vi "Create Dense Cell.vi"() -> ()   [LabVIEW 2020]
uses:
  <vilib>/Analysis/7linalg.llb/Real Transpose Matrix.vi
  <vilib>/Analysis/Matrix/Numeric/Conversions/Array To Matrix - RA2.vi
  <vilib>/Analysis/Matrix/Numeric/Conversions/Matrix To Array - RM.vi
  <vilib>/Analysis/Matrix/NI_Matrix.lvlib
  <vilib>/Analysis/NI_AALPro.lvlib
panel:
  in  "weight path":path
  in  "name":string
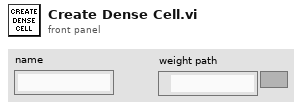
[diagram p1: front panel]
types:
  T1 = typedef "NI_Matrix.lvlib/RealMatrix.ctl" = dbl[][]
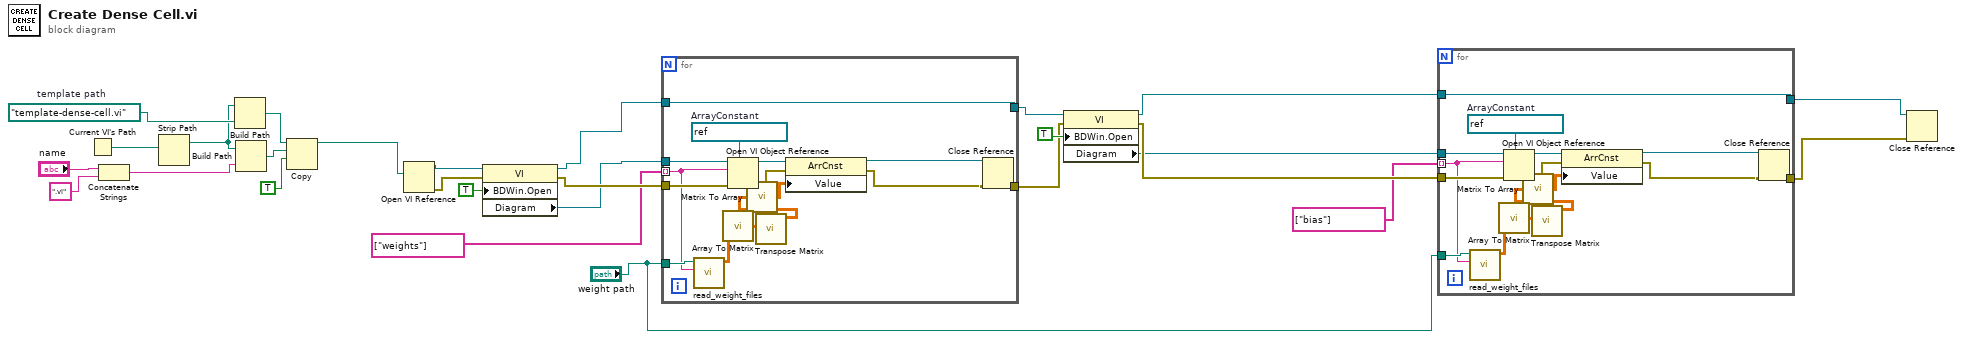
[diagram p0: block diagram]
diagram:
  w15 = path "template-dense-cell.vi"  # template path
  n1 = Current VI's Path() -> (path=w13:path)
  n2 = Concatenate Strings("name", ".vi") -> (w23:string)
  n3 = Strip Path(path=w13) -> (stripped path=w12:path)  [unwired: 1 out]
  n4 = Build Path(base path=w12, name or relative path=w15) -> (appended path=w14:path)
  n5 = Build Path(base path=w12, name or relative path=w23) -> (appended path=w22:path)
  n6 = Copy(9:TRUE, 10:w22, 11:w14) -> (3:w18:path)  [unwired: 2 in, 2 out]
  n7 = Open VI Reference(vi path=w18) -> (vi reference=w20:refnum<vi>, error out=w19:errorcluster)  [unwired: 5 in]
  n8 = property class="VI"(reference=w20, error in=w19, "BDWin.Open"=TRUE) -> (reference out=w16:refnum<vi>, error out=w26:errorcluster, "Diagram"=w17:refnum<vi>)
  n9 = for {
    tunnel: w26 -> [w42]
    tunnel: w17 -> [w41]
    tunnel: string[] ["weights"] -> [w32] mode=indexing
    tunnel: [w36] -> w6
    tunnel: "weight path" -> [w33]
    tunnel: [w37] -> w7
    tunnel: w16 -> [w37]
    w40 = refnum<vi> refnum  # ArrayConstant
    n10 = call "read_weight_files.vi"("weight file name"=w32, "weights path"=w33) -> ("all rows"=w31:dbl[][])  [unwired: 9 in]
    n11 = call-poly <vilib>:"Array To Matrix.vi"("Real 2D Array"=w31) -> ("Real Matrix"=w30:T1)
    n12 = Open VI Object Reference(7:w40, 8:w42, 10:w32, 11:w41) -> (0:w38:errorcluster, 3:w39:refnum<vi>)
    n13 = call-poly <vilib>:"Transpose Matrix.vi"("Input Matrix"=w30) -> ("Matrix Transpose"=w29:T1)  [unwired: 9 in, 1 out]
    n14 = call-poly <vilib>:"Matrix To Array.vi"("Real Matrix"=w29) -> ("Real 2D Array"=w28:dbl[][])
    n15 = property class="ArrCnst"(reference=w39, error in=w38, "Value"=w28) -> (reference out=w35:refnum<vi>, error out=w34:errorcluster)
    n16 = Close Reference(reference=w35, error in (no error)=w34) -> (error out=w36:errorcluster)
  }
  n17 = property class="VI"(reference=w7, error in=w6, "BDWin.Open"=TRUE) -> (reference out=w8:refnum<vi>, error out=w10:errorcluster, "Diagram"=w9:refnum<vi>)
  n18 = for {
    tunnel: w10 -> [w57]
    tunnel: w9 -> [w56]
    tunnel: string[] ["bias"] -> [w47] mode=indexing
    tunnel: [w51] -> w4
    tunnel: "weight path" -> [w48]
    tunnel: [w52] -> w3
    tunnel: w8 -> [w52]
    w55 = refnum<vi> refnum  # ArrayConstant
    n19 = call "read_weight_files.vi"("weight file name"=w47, "weights path"=w48) -> ("all rows"=w46:dbl[][])  [unwired: 9 in]
    n20 = call-poly <vilib>:"Array To Matrix.vi"("Real 2D Array"=w46) -> ("Real Matrix"=w45:T1)
    n21 = Open VI Object Reference(7:w55, 8:w57, 10:w47, 11:w56) -> (0:w53:errorcluster, 3:w54:refnum<vi>)
    n22 = call-poly <vilib>:"Transpose Matrix.vi"("Input Matrix"=w45) -> ("Matrix Transpose"=w44:T1)  [unwired: 9 in, 1 out]
    n23 = call-poly <vilib>:"Matrix To Array.vi"("Real Matrix"=w44) -> ("Real 2D Array"=w43:dbl[][])
    n24 = property class="ArrCnst"(reference=w54, error in=w53, "Value"=w43) -> (reference out=w50:refnum<vi>, error out=w49:errorcluster)
    n25 = Close Reference(reference=w50, error in (no error)=w49) -> (error out=w51:errorcluster)
  }
  n26 = Close Reference(reference=w3, error in (no error)=w4) -> ()  [unwired: 1 out]
